vi "TemperatureRead(SubVI).vi"(5 "CS Configuration 2":T1={"CS Channel"=10, "CS Logic Level"=enum."Active Low"}, 7 "CS Configuration":T1={"CS Channel"=7, "CS Logic Level"=enum."Active High"}, 8 "Error In":errorcluster, 10 "SPI Configuration":T9={"Clock Frequency"=1000000, "Bit Order"=enum."LSb First", "SPI Mode"=enum."Mode 0"}, 11 "LINX Resource":T3={"IO"=enum."Remote", "Interface"=enum."TCP", "LINX Device Config"={"Interface"=enum."TCP", "COM Port"="N/A", "TCP Configuration"={"IP Address"="raspberrypi", "Port"=44301}, "Device Family"=4, "Device ID"=3, "Device Name"="Raspberry Pi 2 Model B\u0000", "TCP Ref"=refnum, "Channels"={"DI"=[7, 11, 12, 13, 15, 16, 18, 22, 29, 31, 32, 33, 35, 36, 37, 38, 40], "DO"=[7, 11, 12, 13, 15, 16, 18, 22, 29, 31, 32, 33, 35, 36, 37, 38, 40], "AI"=[], "AO"=[], "PWM"=[], "QE"=[], "UART"=[0], "I2C 2"=[1], "SPI"=[0], "CAN"=[], "Servo"=[], "AI Ref (V)"=0.0, "AI Resolution (Bits)"=0, "AO Ref (V)"=0.0, "AO Resolution (Bits)"=0}}}) -> (0 "Error Out":errorcluster, 1 "Temp2":string, 2 "Temp1":string, 3 "LINX Resource 2":T3={"IO"=enum."Remote", "Interface"=enum."TCP", "LINX Device Config"={"Interface"=enum."TCP", "COM Port"="N/A", "TCP Configuration"={"IP Address"="raspberrypi", "Port"=44301}, "Device Family"=4, "Device ID"=3, "Device Name"="Raspberry Pi 2 Model B\u0000", "TCP Ref"=refnum, "Channels"={"DI"=[7, 11, 12, 13, 15, 16, 18, 22, 29, 31, 32, 33, 35, 36, 37, 38, 40], "DO"=[7, 11, 12, 13, 15, 16, 18, 22, 29, 31, 32, 33, 35, 36, 37, 38, 40], "AI"=[], "AO"=[], "PWM"=[], "QE"=[], "UART"=[0], "I2C 2"=[1], "SPI"=[0], "CAN"=[], "Servo"=[], "AI Ref (V)"=0.0, "AI Resolution (Bits)"=0, "AO Ref (V)"=0.0, "AO Resolution (Bits)"=0}}}, 4 "Actual Clock Frequency":u32)   [LabVIEW 2017]
uses:
  <vilib>/MakerHub/LINX/Private/Type Defs/Peripherals/SPI/SPI Configuration.ctl
  <vilib>/MakerHub/LINX/Private/Type Defs/Peripherals/SPI/SPI Bit Order.ctl
  <vilib>/MakerHub/LINX/Private/Type Defs/Peripherals/SPI/SPI Mode.ctl
  <vilib>/MakerHub/LINX/Public/Peripherals/SPI/SPI CS Config.ctl
  <vilib>/MakerHub/LINX/Private/Type Defs/Peripherals/SPI/SPI CS Logic Level.ctl
  <vilib>/MakerHub/LINX/Private/Type Defs/LINX Ref.ctl
  <vilib>/MakerHub/LINX/Private/Type Defs/Platform.ctl
  <vilib>/MakerHub/LINX/Private/Type Defs/Interface.ctl
  <vilib>/MakerHub/LINX/Private/Device/Type Defs/LINX Device Config.ctl
  <vilib>/MakerHub/LINX/Private/Device/Type Defs/TCP Config.ctl
  <vilib>/MakerHub/LINX/Private/Device/Type Defs/Channels.ctl
  039def0e-7d84-4ea7-8810-6bd0fda254d9.vi
  40574007-0335-4ab6-9cc9-f30f3a1ac072.vi
  <vilib>/MakerHub/LINX/LMH-LINX.lvlib
  <vilib>/MakerHub/LINX/Private/Device/Device.lvlib
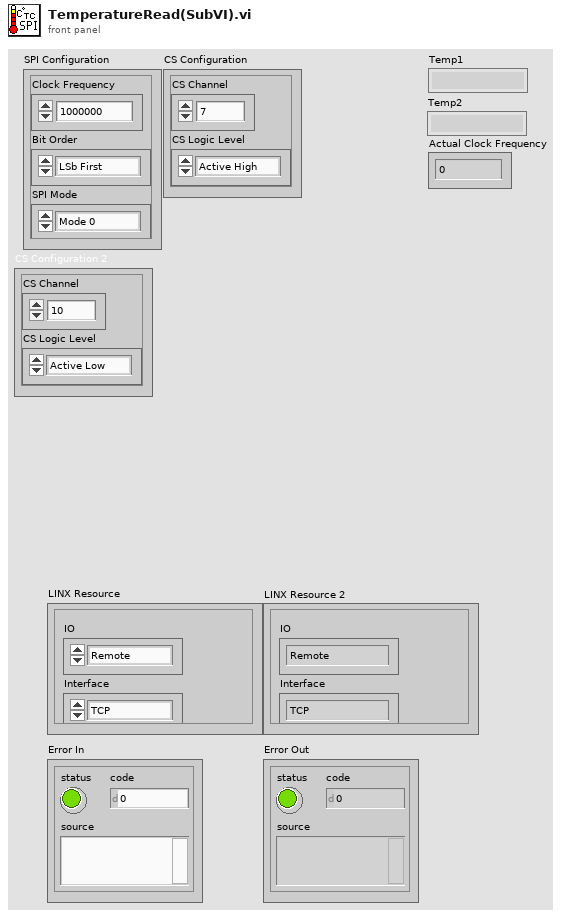
[diagram p1: front panel]
types:
  T1 = typedef "LMH-LINX.lvlib/SPI CS Config.ctl" = cluster{"CS Channel":u8, "CS Logic Level":T2}
  T2 = typedef "LMH-LINX.lvlib/SPI CS Logic Level.ctl" = enum8{"Active Low", "Active High"}
  T3 = typedef "LMH-LINX.lvlib/LINX Ref.ctl" = cluster{"IO":T4, "Interface":T5, "LINX Device Config":T6}
  T4 = typedef "LMH-LINX.lvlib/Platform.ctl" = enum16{"Remote", "Local"}
  T5 = typedef "LMH-LINX.lvlib/Interface.ctl" = enum16{"Serial", "TCP"}
  T6 = typedef "LMH-LINX.lvlib/Device.lvlib/LINX Device Config.ctl" = cluster{"Interface":T5, "COM Port":refnum<visa-resource-name>, "TCP Configuration":T7, "Device Family":u8, "Device ID":u8, "Device Name":string, "TCP Ref":refnum<k5>, "Channels":T8}
  T7 = typedef "LMH-LINX.lvlib/Device.lvlib/TCP Config.ctl" = cluster{"IP Address":string, "Port":u16}
  T8 = typedef "LMH-LINX.lvlib/Channels.ctl" = cluster{"DI":u8[], "DO":u8[], "AI":u8[], "AO":u8[], "PWM":u8[], "QE":u8[], "UART":u8[], "I2C 2":u8[], "SPI":u8[], "CAN":u8[], "Servo":u8[], "AI Ref (V)":dbl, "AI Resolution (Bits)":u8, "AO Ref (V)":dbl, "AO Resolution (Bits)":u8}
  T9 = typedef "LMH-LINX.lvlib/SPI Configuration.ctl" = cluster{"Clock Frequency":u32, "Bit Order":T10, "SPI Mode":T11}
  T10 = typedef "LMH-LINX.lvlib/SPI Bit Order.ctl" = enum8{"LSb First", "MSb First"}
  T11 = typedef "LMH-LINX.lvlib/SPI Mode.ctl" = enum8{"Mode 0", "Mode 1", "Mode 2", "Mode 3"}
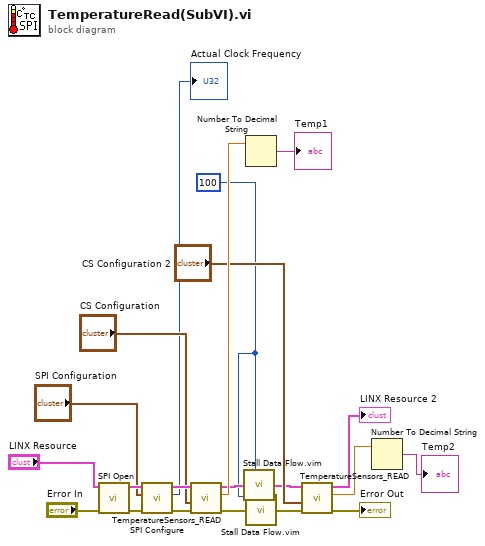
[diagram p0: block diagram]
diagram:
  w1 = u32 100 ("milliseconds to wait")
  n1 = call <vilib>:"SPI Open.vi"("Error In"="Error In", "LINX Resource"="LINX Resource") -> ("Error Out"=w20:errorcluster, "LINX Resource"=w21:T3)  [unwired: 8 in]
  n2 = call <vilib>:"SPI Configure.vi"("Error In"=w20, "SPI Configuration"="SPI Configuration", "LINX Resource"=w21) -> ("Error Out"=w15:errorcluster, "Actual Clock Frequency"=→"Actual Clock Frequency":u32, "LINX Resource"=w16:T3)  [unwired: 6 in]
  n3 = call "TemperatureSensors_READ.vi"("Error IN"=w15, "CS Configuration"="CS Configuration", "LINX Resource IN"=w16) -> ("Error OUT"=w3:errorcluster, "Temperature [°C]"=w13:dbl, "LINX Resource OUT"=w5:T3)  [unwired: 3 in, 3 out]
  n4 = call "Stall Data Flow.vim"("value in"=w5, "milliseconds to wait"=w1) -> ("value out"=w4:T3)  [unwired: 1 out]
  n5 = Number To Decimal String(number=w13) -> (decimal integer string=→"Temp1":string)  [unwired: 1 in]
  n6 = call "Stall Data Flow.vim"("value in"=w3, "milliseconds to wait"=w1) -> ("value out"=w2:errorcluster)  [unwired: 1 out]
  n7 = call "TemperatureSensors_READ.vi"("Error IN"=w2, "CS Configuration"="CS Configuration 2", "LINX Resource IN"=w4) -> ("Error OUT"=→"Error Out":errorcluster, "Temperature [°C]"=w8:dbl, "LINX Resource OUT"=→"LINX Resource 2":T3)  [unwired: 3 in, 3 out]
  n8 = Number To Decimal String(number=w8) -> (decimal integer string=→"Temp2":string)  [unwired: 1 in]
